vi "Actor Core.vi"(8 "error in":errorcluster, 11 "Business Logic in":refnum<class "Business Logic.lvclass">) -> (0 "error out":errorcluster, 3 "Actor out":refnum<class "Actor.lvclass">)   [LabVIEW 2020, in "Business Logic.lvlib" / "Business Logic.lvclass"]
doc: "(<B>Filename</B>: Actor Framework.lvlib:Actor.lvclass:Actor Core.vi)\n\nReceives messages to the actor, reacts to them, and initiates any error handling that may shut the actor down.\n\nDescendant classes may override this VI to append parallel tasks for the actor to complete while it handles messages. Overrides use the Call Parent Class Method node."
uses:
  Business Logic.lvclass
  Business Logic.lvclass/Business Logic.ctl
  <vilib>/ActorFramework/Actor/Actor.lvclass
  C:/Program Files (x86)/National Instruments/LabVIEW 2020/vi.lib/ActorFramework/Actor/Actor.lvclass
  D:/Storage/Source Code/Clase AF/ClaseAF/09 Controls and Indicators AF/Business Logic/Business Logic/Business Logic.lvclass
  Controls/Controls.lvclass
  Indicators/Indicators.lvclass
  Controls Messages/Set HW ID Msg/Set HW ID Msg.lvclass
  D:/Storage/Source Code/Clase AF/ClaseAF/09 Controls and Indicators AF/Controls/Controls.lvclass
  D:/Storage/Source Code/Clase AF/ClaseAF/09 Controls and Indicators AF/Indicators/Indicators.lvclass
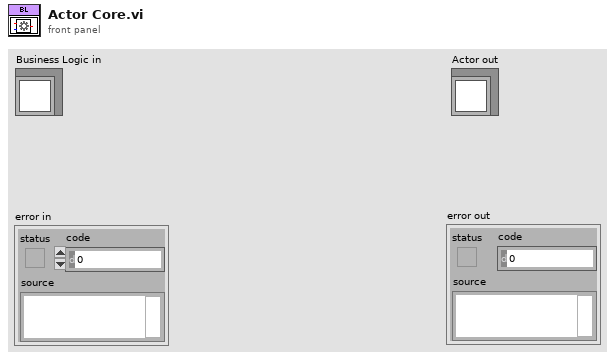
[diagram p1: front panel]
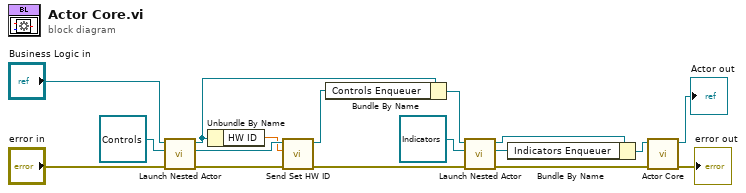
[diagram p0: block diagram]
diagram:
  n1 = call <vilib>:"Launch Nested Actor.vi"("error in (no error)"="error in", "Nested Actor"=refnum<class "Controls.lvclass"> refnum ("Controls.lvlib:Controls.lvclass"), "Caller Actor in"="Business Logic in") -> ("error out"=w4:errorcluster, "Nested Actor's Enqueuer"=w6:refnum<class "Message Enqueuer.lvclass">, "Caller Actor out"=w2:refnum<class "Business Logic.lvclass">)  [unwired: 6 in]
  n2 = Unbundle By Name(w2) -> ("HW ID"=w1:dbl)
  n3 = call "Send Set HW ID.vi"("error in (no error)"=w4, "HW ID"=w1, "Message Enqueuer"=w6) -> ("error out"=w3:errorcluster, "Message Enqueuer out"=w5:refnum<class "Message Enqueuer.lvclass">)  [unwired: 7 in]
  n4 = Bundle By Name(cluster=w2, "Controls Enqueuer"=w5) -> (w9:refnum<class "Business Logic.lvclass">)
  n5 = call <vilib>:"Launch Nested Actor.vi"("error in (no error)"=w3, "Nested Actor"=refnum<class "Indicators.lvclass"> refnum ("Indicators.lvlib:Indicators.lvclass"), "Caller Actor in"=w9) -> ("error out"=w13:errorcluster, "Nested Actor's Enqueuer"=w7:refnum<class "Message Enqueuer.lvclass">, "Caller Actor out"=w12:refnum<class "Business Logic.lvclass">)  [unwired: 6 in]
  n6 = Bundle By Name(cluster=w12, "Indicators Enqueuer"=w7) -> (w8:refnum<class "Business Logic.lvclass">)
  n7 = call-parent "Actor Core.vi"("error in"=w13, "Actor in"=w8) -> ("error out"=→"error out":errorcluster, "Actor out"=→"Actor out":refnum<class "Actor.lvclass">)  [unwired: 8 in]
